vi "array -- poor man hash table -- cluster keyed -- test.vi"() -> ()   [LabVIEW 2012]
uses:
  hash action control.ctl
  torque -- hash key.ctl
  hash status control.ctl
panel:
  out "index":i32
  out "found?":bool
  in  "key table":T1[](array[typedef])
  in  "hash key":T1
  in  "hash action":T2
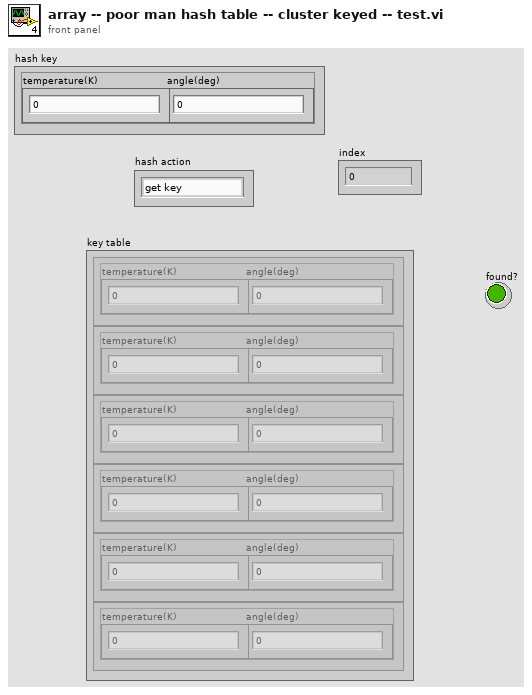
[diagram p1: front panel]
types:
  T1 = typedef "torque -- hash key.ctl" = cluster{"temperature(K)":dbl, "angle(deg)":dbl}
  T2 = typedef "hash action control.ctl" = enum16{"get key", "new key", "--void", "delete key", "delete all", "create key if not found", "--delete if found", "--create if not found"}
  T3 = typedef "hash status control.ctl" = enum16{"exists", "does not exists"}
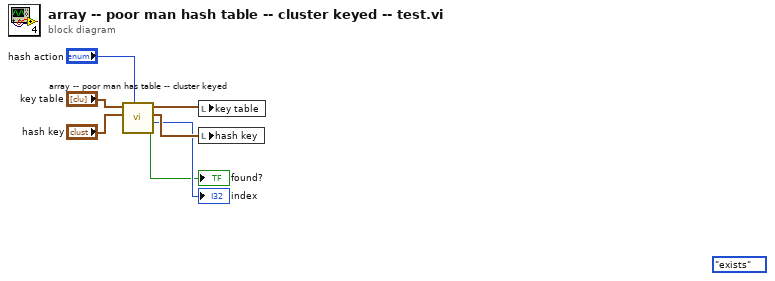
[diagram p0: block diagram]
diagram:
  (unwired) hash_status_control."exists" ("hash status")
  n1 = call "array -- poor man has table -- cluster keyed .vi"("hash action"="hash action", "hash key"="hash key", "key table"="key table") -> ("found?"=→"found?":bool, "index"=→"index":i32, "hash key OUT"=w5:T1, "Key table OUT"=w6:T1[])  [unwired: 5 in]
  n2 = local write "key table"(w6) -> ()
  n3 = local write "hash key"(w5) -> ()
